vi "Plot Helper.vi"   [LabVIEW 2020, in "2D Compass Datatype.lvclass"]
doc: "Graphs vectors that emanate from the center origin in a compass plot. Multiple references to this VI generate multiple plots on the same graph."
uses:
  <vilib>/Math Plots/2D Math Plots/2D Compass/2D Compass Datatype/2D Compass Datatype.lvclass
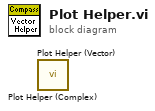
[diagram p0: block diagram]
diagram:
  n1 = call <vilib>:"Plot Helper (Complex).vi"() -> ()  [unwired: 10 in, 2 out]
  n2 = call <vilib>:"Plot Helper (Vector).vi"() -> ()  [unwired: 10 in, 2 out]
